vi "GetSetTemplateVersions.vi"() -> ()   [LabVIEW 2020]
panel:
  out "error out":errorcluster
  in  "error in":errorcluster
  in  "error in (no error)":errorcluster
  out "Array":T1(array[cluster])
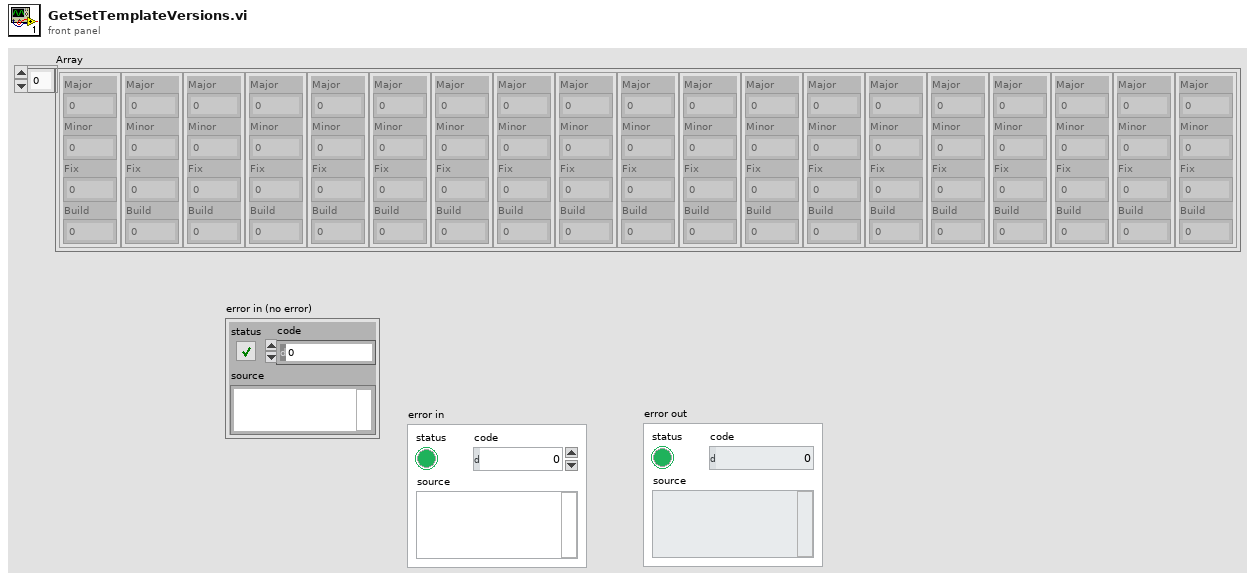
[diagram p1: front panel]
types:
  T1 = cluster{"Major":u16, "Minor":u16, "Fix":u16, "Build":u16}[]
  T2 = cluster{"Major":i32, "Minor":u16, "Fix":u16, "Build":i32}
  T3 = cluster{"Major":u16, "Minor":u16, "Fix":u16, "Build":u16}
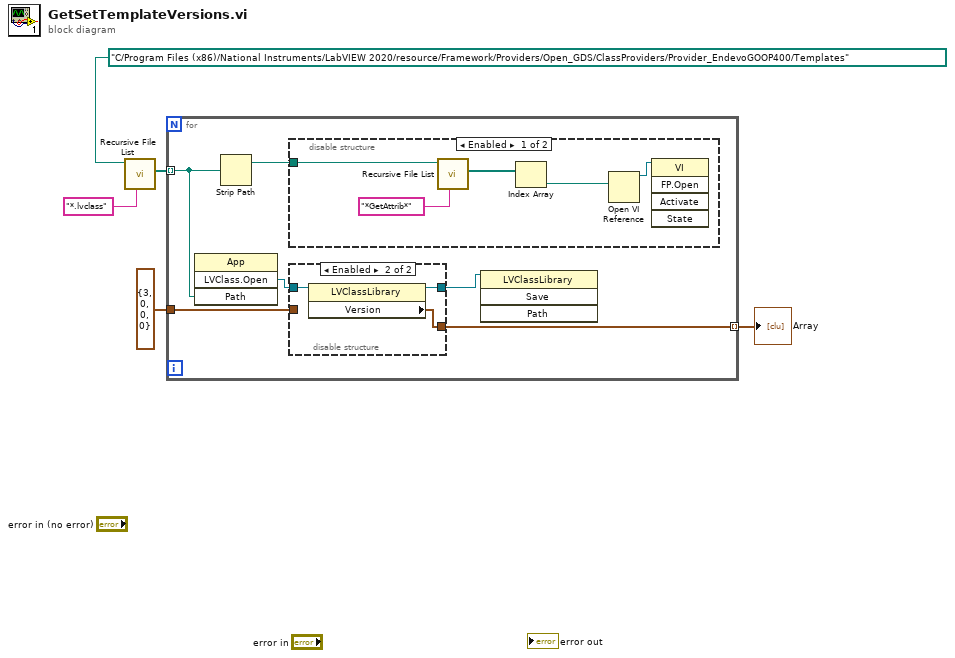
[diagram p0: block diagram]
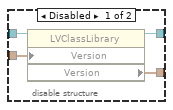
[diagram p2: hidden frame]
diagram:
  n1 = call <vilib>:"Recursive File List.vi"("pattern"="*.lvclass", "Folder Path"=path "C:/Program Files (x86)/National Instruments/LabVIEW 2020/resource/Framework/Providers/Open_GDS/ClassProviders/Provider_EndevoGOOP400/Templates" ("Folder to Search")) -> ("All Files in Dir"=w3:path[])  [unwired: 5 in, 4 out]
  n2 = for {
    tunnel: w3 -> [w9] mode=indexing
    tunnel: [w10] -> w2 mode=indexing
    tunnel: T2 {"Major"=3, "Minor"=0, "Fix"=0, "Build"=0} ("Version") -> [w7]
    n3 = invoke class="App" method="LVClass.Open"("Path"=w9) -> ("LVClass.Open"=w11:refnum<vi>)  [unwired: 3 in, 3 out]
    n4 = Strip Path(path=w9) -> (stripped path=w8:path)  [unwired: 1 out]
    n5 = disable-structure shown="Enabled" {
      disable-tunnel: w8 -> [w22 _]
      frame Enabled {
        n6 = call <vilib>:"Recursive File List.vi"("pattern"="*GetAttrib*", "Folder Path"=w22) -> ("All Files in Dir"=w20:path[])  [unwired: 5 in, 4 out]
        n7 = Index Array(array=w20) -> (element=w19:path)  [unwired: 1 in]
        n8 = Open VI Reference(vi path=w19) -> (vi reference=w21:refnum<vi>)  [unwired: 5 in, 1 out]
        n9 = invoke class="VI" method="FP.Open"(reference=w21) -> ()  [unwired: 4 in, 5 out]
      }
      frame Disabled {
      }
    }
    n10 = disable-structure shown="Enabled" {
      disable-tunnel: w11 -> [w15 w18]
      disable-tunnel: [w14 w17] -> w10
      disable-tunnel: w7 -> [w13 _]
      disable-tunnel: [w12 w16] -> w6
      frame Disabled {
        n11 = property class="LVClassLibrary"(reference=w15, "Version"=w13) -> (reference out=w12:refnum<vi>, "Version"=w14:T3)  [unwired: 1 in, 1 out]
      }
      frame Enabled {
        n12 = property class="LVClassLibrary"(reference=w18) -> (reference out=w16:refnum<vi>, "Version"=w17:T3)  [unwired: 1 in, 1 out]
      }
    }
    n13 = invoke class="LVClassLibrary" method="Save"(reference=w6) -> ()  [unwired: 3 in, 4 out]
  }
  "Array" <- w2
